vi "Teleop.vi"(10 "Match Info":T1={"Autonomous Elapsed Seconds"=0.0, "TeleOp Elapsed Seconds"=0.0, "Disabled Elapsed Seconds"=0.0, "Visited Autonomous"=FALSE, "Visited TeleOp"=FALSE, "Visited Disabled"=FALSE, "Autonomous Settings"={"Autonomous Style"=enum."Independent", "VI Refnum"=refnum}}, 11 "Call Context":T2) -> ()   [LabVIEW 2011]
doc: "This VI is called for each TeleOp packet received from the DS where the robot is not disabled. It is often used to read from the joysticks and update I/O or to update setpoints for timed control loops. It should complete and return within 20 milliseconds or it may miss DS packets."
uses:
  <vilib>/Rock Robotics/WPI/DriverStation/WPI_DriverStationDerivedRobotMode.ctl
  <vilib>/Rock Robotics/WPI/DriverStation/WPI_DriverStationMatch Info.ctl
  Robot Global Data.vi
panel:
  out "PreviousDriverControlMode":bool
  in  "Motor 6":dbl=0.25
  in  "Motor 5":dbl=0.7
  in  "Motor 4.5":dbl=0.5
  in  "Motor 4":dbl=0.35
  in  "Motor 3.5":dbl=0.3
  in  "Speed 6":dbl
  in  "Speed 5":dbl=1394.7264
  in  "Speed 4.5":dbl=1080.1728
  in  "Speed 4":dbl=963.1296
  in  "Speed 3.5":dbl
  # "Front key middle basket"
  # "Front key high basket"
  # "Back key high basket"
  # "Front bumper touches the barrier high basket"
  # "Fender, low basket"
  # "Speed by encoder"
  # "Motor absolute value"
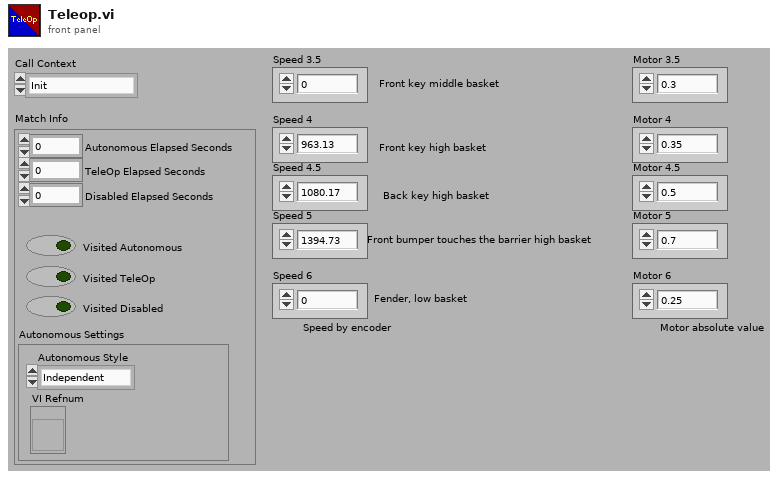
[diagram p1: front panel]
types:
  T1 = typedef "WPI_DriverStationMatch Info.ctl" = cluster{"Autonomous Elapsed Seconds":dbl, "TeleOp Elapsed Seconds":dbl, "Disabled Elapsed Seconds":dbl, "Visited Autonomous":bool, "Visited TeleOp":bool, "Visited Disabled":bool, "Autonomous Settings":cluster{"Autonomous Style":enum16{"Iterative", "Independent"}, "VI Refnum":refnum<vi>}}
  T2 = typedef "WPI_DriverStationDerivedRobotMode.ctl" = enum16{"Init", "Execute", "Stop"}
  T3 = typedef "WPI_JoystickDevRef.ctl" = cluster{"Device":T4}
  T4 = typedef "WPI_JoystickDeviceEnum.ctl" = enum16{"USB 1", "USB 2", "USB 3", "USB 4", "Kinect 1", "Kinect 2"}
  T5 = typedef "WPI_JoystickButtonState.ctl" = cluster{"Button 1":bool, "Button 2":bool, "Button 3":bool, "Button 4":bool, "Button 5":bool, "Button 6":bool, "Button 7":bool, "Button 8":bool, "Button 9":bool, "Button 10":bool, "Button 11":bool, "Button 12":bool}
  T6 = cluster{"axis 1 (x)":dbl, "axis 2 (y)":dbl, "axis 3 (throttle)":dbl, "axis 4":dbl, "axis 5":dbl, "axis 6":dbl}
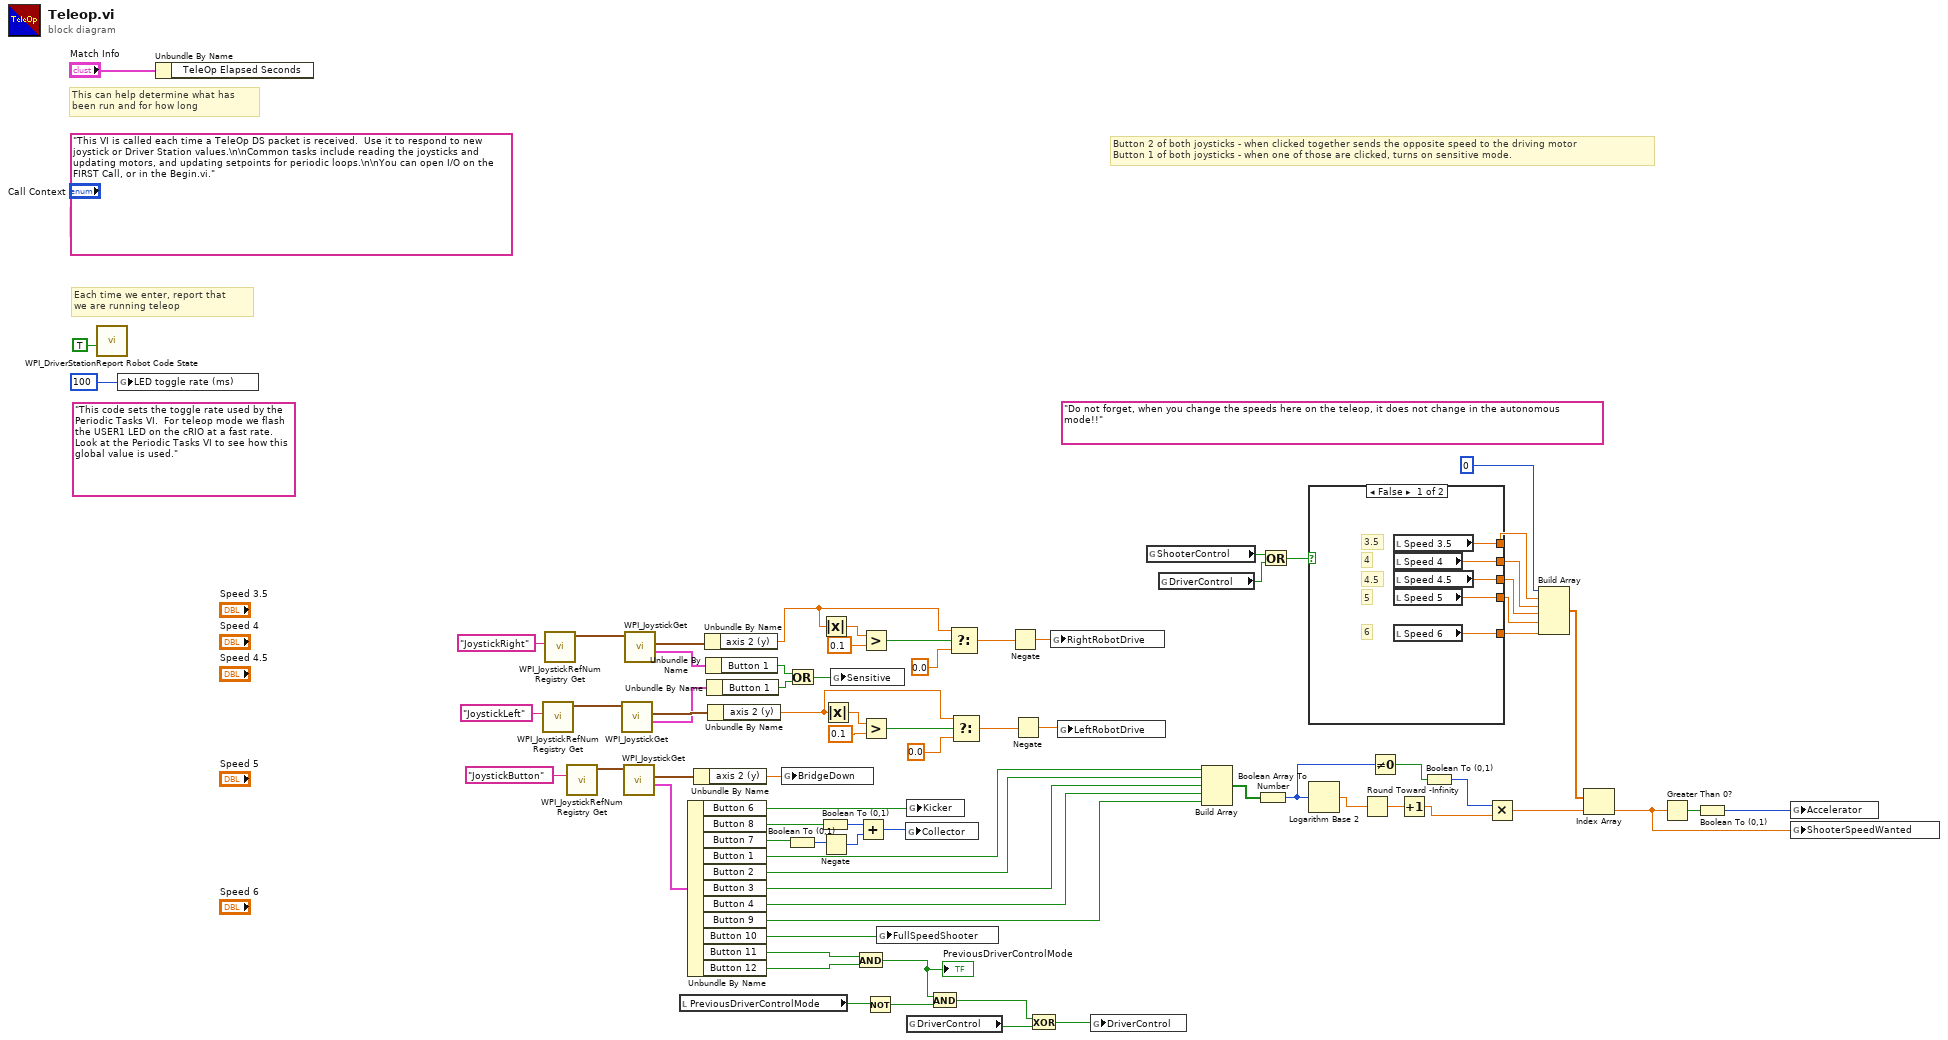
[diagram p0: block diagram]
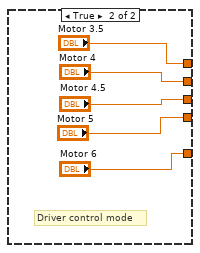
[diagram p2: hidden frame]
diagram:
  (unwired) "Do not forget, when you change the speeds here on the teleop, it does not change in the autonomous mode!!"
  (unwired) "This code sets the toggle rate used by the Periodic Tasks VI.  For teleop mode we flash the USER1 LED on the cRIO at a fast rate.  Look at the Periodic Tasks VI to see how this global value is used."
  (unwired) "This VI is called each time a TeleOp DS packet is received.  Use it to respond to new joystick or Driver Station values.\n\nCommon tasks include reading the joysticks and updating motors, and updating setpoints for periodic loops.\n\nYou can open I/O on the FIRST Call, or in the Begin.vi."
  # "Button 2 of both joysticks - when clicked together sends the opposite speed to the driving motor\nButton 1 of both joysticks - when one of those are clicked, turns on sensitive mode."
  # "Each time we enter, report that\nwe are running teleop"
  # "Use to differentiate between\nFirst, Last, and Intermediate calls"
  # "This can help determine what has\nbeen run and for how long"
  n1 = call <vilib>:"WPI_DriverStationReport Robot Code State.vi"("TeleOp"=TRUE ("Autonomous")) -> ()  [unwired: 10 in, 1 out]
  n2 = global write "Robot Global Data.vi" "LED toggle rate (ms)"(u32 100 ("LED ms toggle rate")) -> ()
  n3 = Unbundle By Name("Match Info") -> ()  [unwired: 1 out]
  n4 = call <vilib>:"WPI_JoystickRefNum Registry Get.vi"("refnum name"="JoystickLeft") -> ("JoystickDevRef"=w71:T3)  [unwired: 9 in, 1 out]
  n5 = call <vilib>:"WPI_JoystickRefNum Registry Get.vi"("refnum name"="JoystickRight") -> ("JoystickDevRef"=w70:T3)  [unwired: 9 in, 1 out]
  n6 = call <vilib>:"WPI_JoystickRefNum Registry Get.vi"("refnum name"="JoystickButton") -> ("JoystickDevRef"=w50:T3)  [unwired: 9 in, 1 out]
  n7 = call <vilib>:"WPI_JoystickGet.vi"("JoystickDevRef"=w71) -> ("Buttons"=w67:T5, "Axes"=w69:T6)  [unwired: 4 in, 1 out]
  n8 = call <vilib>:"WPI_JoystickGet.vi"("JoystickDevRef"=w50) -> ("Buttons"=w49:T5, "Axes"=w43:T6)  [unwired: 4 in, 1 out]
  n9 = call <vilib>:"WPI_JoystickGet.vi"("JoystickDevRef"=w70) -> ("Buttons"=w47:T5, "Axes"=w66:T6)  [unwired: 4 in, 1 out]
  n10 = local read "PreviousDriverControlMode"() -> (w20:bool)
  n11 = Unbundle By Name(w49) -> ("Button 6"=w5:bool, "Button 8"=w7:bool, "Button 7"=w6:bool, "Button 1"=w29:bool, "Button 2"=w28:bool, "Button 3"=w27:bool, "Button 4"=w26:bool, "Button 9"=w14:bool, "Button 10"=w13:bool, "Button 11"=w23:bool, "Button 12"=w24:bool)
  n12 = Unbundle By Name(w43) -> ("axis 2 (y)"=w12:dbl)
  n13 = Unbundle By Name(w66) -> ("axis 2 (y)"=w62:dbl)
  n14 = Unbundle By Name(w47) -> ("Button 1"=w54:bool)
  n15 = Unbundle By Name(w67) -> ("Button 1"=w53:bool)
  n16 = Unbundle By Name(w69) -> ("axis 2 (y)"=w57:dbl)
  n17 = global write "Robot Global Data.vi" "BridgeDown"(w12) -> ()
  n18 = Boolean To (0,1)(Boolean=w6) -> (0, 1=w11:i16)
  n19 = Or(x=w54, y=w53) -> (x .or. y?=w52:bool)
  n20 = Boolean To (0,1)(Boolean=w7) -> (0, 1=w8:i16)
  n21 = Absolute Value(x=w62) -> (abs(x)=w65:dbl)
  n22 = Negate(x=w11) -> (-x=w10:i16)
  n23 = Absolute Value(x=w57) -> (abs(x)=w61:dbl)
  n24 = global write "Robot Global Data.vi" "Sensitive"(w52) -> ()
  n25 = And(x=w23, y=w24) -> (x .and. y?=w18:bool)
  "PreviousDriverControlMode" <- w18
  n26 = Add(x=w8, y=w10) -> (x+y=w9:i16)
  n27 = Greater?(x=w65, y=0.1 ("x")) -> (0:w63:bool)
  n28 = Greater?(x=w61, y=0.1 ("x")) -> (0:w59:bool)
  n29 = Not(x=w20) -> (.not. x?=w19:bool)
  n30 = global write "Robot Global Data.vi" "FullSpeedShooter"(w13) -> ()
  n31 = global write "Robot Global Data.vi" "Collector"(w9) -> ()
  n32 = global write "Robot Global Data.vi" "Kicker"(w5) -> ()
  n33 = global read "Robot Global Data.vi" "DriverControl"() -> (w22:bool)
  n34 = And(x=w18, y=w19) -> (x .and. y?=w17:bool)
  n35 = Select(t=w62, s=w63, f=0.0) -> (s? t:f=w55:dbl)
  n36 = Select(t=w57, s=w59, f=0.0) -> (s? t:f=w56:dbl)
  n37 = Negate(x=w55) -> (-x=w46:dbl)
  n38 = Negate(x=w56) -> (-x=w45:dbl)
  n39 = Exclusive Or(1:w22, 2:w17) -> (0:w21:bool)
  n40 = global write "Robot Global Data.vi" "RightRobotDrive"(w46) -> ()
  n41 = global write "Robot Global Data.vi" "LeftRobotDrive"(w45) -> ()
  n42 = global write "Robot Global Data.vi" "DriverControl"(w21) -> ()
  n43 = global read "Robot Global Data.vi" "ShooterControl"() -> (w1:bool)
  n44 = global read "Robot Global Data.vi" "DriverControl"() -> (w2:bool)
  n45 = Build Array(w29, w28, w27, w26, w14) -> (w25:bool[])
  n46 = Boolean Array To Number(Boolean array=w25) -> (number=w36:u32)
  n47 = Or(x=w1, y=w2) -> (x .or. y?=w3:bool)
  n48 = case shown="False" w3 {
    tunnel: [w80 "Motor 6"] -> w15
    tunnel: [w79 "Motor 5"] -> w4
    tunnel: [w78 "Motor 4.5"] -> w32
    tunnel: [w77 "Motor 4"] -> w31
    tunnel: [w76 "Motor 3.5"] -> w30
    frame False {
      # "4"
      # "6"
      # "5"
      # "4.5"
      # "3.5"
      n49 = local read "Speed 3.5"() -> (w76:dbl)
      n50 = local read "Speed 4"() -> (w77:dbl)
      n51 = local read "Speed 4.5"() -> (w78:dbl)
      n52 = local read "Speed 5"() -> (w79:dbl)
      n53 = local read "Speed 6"() -> (w80:dbl)
    }
    frame True {
      # "Driver control mode"
    }
  }
  n54 = Logarithm Base 2(1:w36) -> (0:w35:dbl)
  n55 = Round Toward -Infinity(1:w35) -> (0:w34:dbl)
  n56 = Not Equal To 0?(x=w36) -> (x != 0?=w37:bool)
  n57 = Increment(x=w34) -> (x+1=w33:dbl)
  n58 = Boolean To (0,1)(Boolean=w37) -> (0, 1=w40:i16)
  n59 = Multiply(x=w40, y=w33) -> (x*y=w39:dbl)
  n60 = Build Array(0, w30, w31, w32, w4, w15) -> (w41:dbl[])
  n61 = Index Array(array=w41, index=w39) -> (element=w16:dbl)
  n62 = Greater Than 0?(x=w16) -> (x > 0?=w38:bool)
  n63 = Boolean To (0,1)(Boolean=w38) -> (0, 1=w48:i16)
  n64 = global write "Robot Global Data.vi" "Accelerator"(w48) -> ()
  n65 = global write "Robot Global Data.vi" "ShooterSpeedWanted"(w16) -> ()
